vi "Read Frame (Text).vi"(8 "error in (no error)":errorcluster, 9 "timeout (1000 ms)":i32=1000, 11 "Connection.WS":refnum<class "Connection.WS.lvclass">) -> (0 "error out":errorcluster, 1 "timed out":bool, 2 "Text":string, 3 "Connection.WS":refnum<class "Connection.WS.lvclass">, 4 "connected":bool, 5 "isTextFrame?":bool)   [LabVIEW 2013, in "Connection.WS_GOSPL.lvlib" / "Connection.WS.lvclass"]
uses:
  Connection.WS.lvclass
  Websocket Frame Type -- ring.ctl
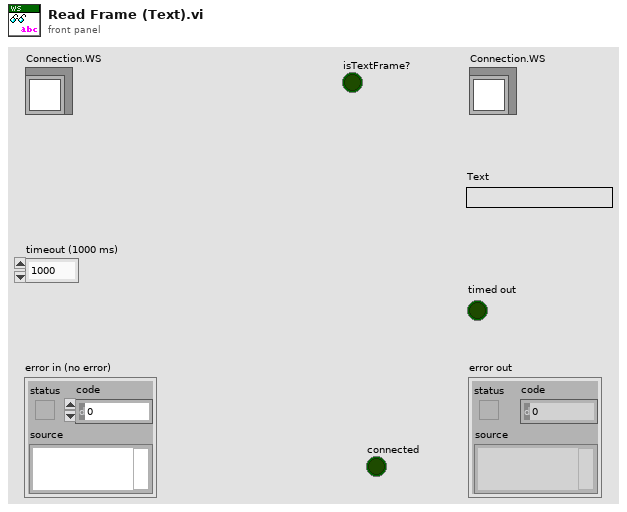
[diagram p1: front panel]
types:
  T1 = typedef "Connection.WS_GOSPL.lvlib/Connection.WS.lvclass/Websocket Frame Type -- ring.ctl" = u8
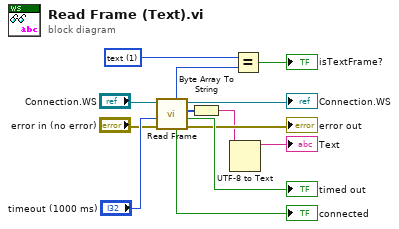
[diagram p0: block diagram]
diagram:
  w4 = T1 1 items=["continuation"=0, "text"=1, "binary"=2, "close"=8, "ping"=9, "pong"=10] ("x")
  n1 = call "Read Frame.vi"("error in (no error)"="error in (no error)", "timeout (1000 ms)"="timeout (1000 ms)", "Connection.WS"="Connection.WS") -> ("error out"=→"error out":errorcluster, "timed out"=→"timed out":bool, "Bytes"=w6:u8[], "Connection.WS"=→"Connection.WS":refnum<class "Connection.WS.lvclass">, "connected"=→"connected":bool, "Frame Type"=w5:T1)  [unwired: 3 in]
  n2 = Byte Array To String(unsigned byte array=w6) -> (string=w2:string)
  n3 = UTF-8 to Text(11:w2) -> (3:→"Text":string)  [unwired: 1 in, 1 out]
  n4 = Equal?(x=w4, y=w5) -> (x = y?=→"isTextFrame?":bool)
